vi "Autonomous Independent.vi"   [LabVIEW 2014]
doc: "This VI is called when autonomous begins, and will automatically be terminated when autonomous ends. You can carry out timed or sensor driven robot movement independently without needing to return to the caller."
uses:
  <vilib>/Rock Robotics/WPI/Joystick/WPI_JoystickGetSetRefNum.vi
panel:
  # "Be sure to right-click and choose Data Operations>>Make Current Value default if you want to save the array values with the VI"
types:
  T1 = typedef "WPI_JoystickDevRef.ctl" = cluster{"Device":T2}
  T2 = typedef "WPI_JoystickDeviceEnum.ctl" = enum16{"USB 0", "USB 1", "USB 2", "USB 3", "USB 4", "USB 5"}
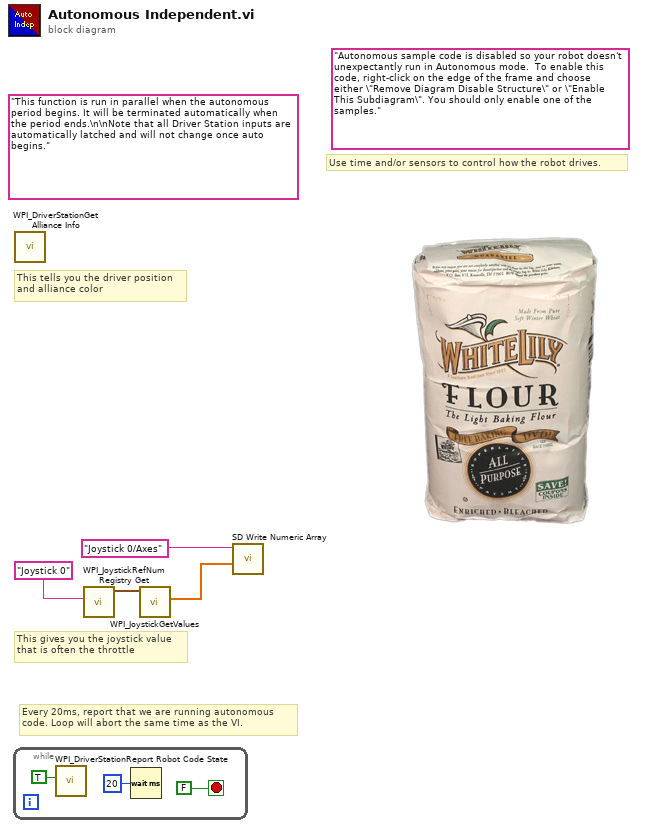
[diagram p0: block diagram]
diagram:
  (unwired) "Autonomous sample code is disabled so your robot doesn't unexpectantly run in Autonomous mode.  To enable this code, right-click on the edge of the frame and choose either \"Remove Diagram Disable Structure\" or \"Enable This Subdiagram\". You should only enable one of the samples."
  (unwired) "This function is run in parallel when the autonomous period begins. It will be terminated automatically when the period ends.\n\nNote that all Driver Station inputs are automatically latched and will not change once auto begins."
  # "Every 20ms, report that we are running autonomous\ncode. Loop will abort the same time as the VI."
  # "This gives you the joystick value\nthat is often the throttle"
  # "Use time and/or sensors to control how the robot drives."
  # "This tells you the driver position\nand alliance color"
  n1 = while {
    stop <- FALSE stop-if-true
    n2 = call <vilib>:"WPI_DriverStationReport Robot Code State.vi"("Autonomous"=TRUE) -> ()  [unwired: 10 in, 1 out]
    n3 = Wait (ms)(milliseconds to wait=u32 20) -> ()  [unwired: 1 out]
  }
  n4 = call <vilib>:"WPI_DriverStationGet Alliance Info.vi"() -> ()  [unwired: 12 out]
  n5 = call <vilib>:"WPI_JoystickRefNum Registry Get.vi"("refnum name"="Joystick 0") -> ("JoystickDevRef"=w3:T1)  [unwired: 1 in, 9 out]
  n6 = call <vilib>:"WPI_JoystickGetValues.vi"("JoystickDevRef"=w3) -> ("Axes"=w1:dbl[])  [unwired: 6 in, 4 out]
  n7 = call <vilib>:"SD Write Numeric Array.vi"("Numeric Array"=w1, "Name"="Joystick 0/Axes") -> ()  [unwired: 8 in, 2 out]
